vi "getPIDRawRead.vi"(11 "PIDController in":refnum<class "PIDController.lvclass">) -> (2 "PIDRawRead":dbl, 3 "PIDController out":refnum<class "PIDController.lvclass">)   [LabVIEW 2025, in "PIDController.lvclass"]
uses:
  PIDController.lvclass/PIDController.ctl
  PIDController.lvclass
panel:
  out "translatedPIDOutput":dbl
  in  "sensorValue":dbl
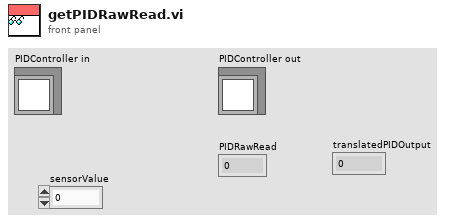
[diagram p1: front panel]
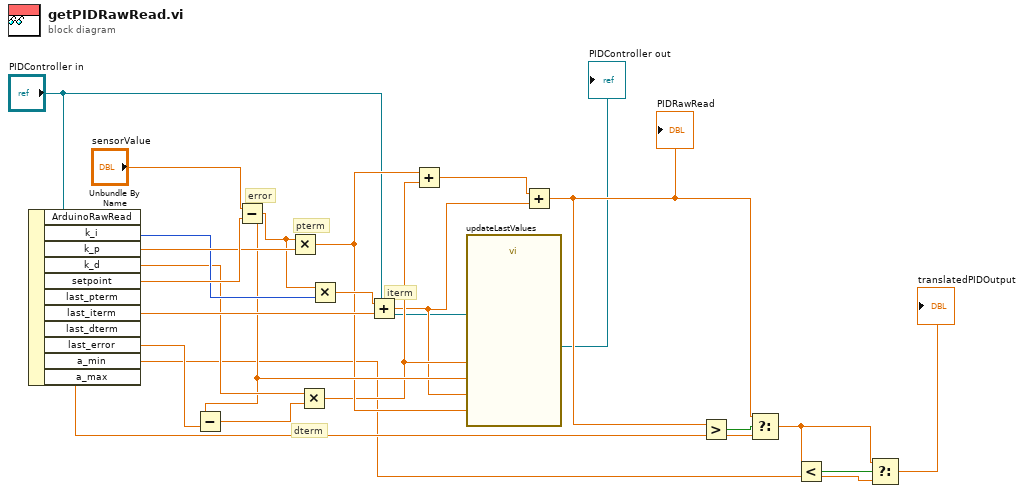
[diagram p0: block diagram]
diagram:
  # "dterm"
  # "iterm"
  # "error"
  # "pterm"
  n1 = Unbundle By Name("PIDController in") -> ("k_i"=w19:u16, "k_p"=w21:dbl, "k_d"=w17:dbl, "setpoint"=w22:dbl, "last_iterm"=w20:dbl, "last_error"=w15:dbl, "a_min"=w4:dbl, "a_max"=w7:dbl)  [unwired: 3 out]
  n2 = Subtract(x="sensorValue", y=w22) -> (x-y=w14:dbl)
  n3 = Subtract(x=w14, y=w15) -> (x-y=w16:dbl)
  n4 = Multiply(x=w14, y=w21) -> (x*y=w13:dbl)
  n5 = Multiply(x=w17, y=w16) -> (x*y=w12:dbl)
  n6 = Multiply(x=w14, y=w19) -> (x*y=w18:dbl)
  n7 = Add(x=w18, y=w20) -> (x+y=w11:dbl)
  n8 = Add(x=w13, y=w12) -> (x+y=w10:dbl)
  n9 = call "updateLastValues.vi"("last_iterm"=w11, "last_dterm"=w12, "last_error"=w14, "last_pterm"=w13, "PIDController in"="PIDController in") -> ("PIDController out"=→"PIDController out":refnum<class "PIDController.lvclass">)  [unwired: 5 in, 1 out]
  n10 = Add(x=w10, y=w11) -> (x+y=w8:dbl)
  "PIDRawRead" <- w8
  n11 = Greater?(x=w8, y=w7) -> (0:w9:bool)
  n12 = Select(t=w8, s=w9, f=w7) -> (s? t:f=w5:dbl)
  n13 = Less?(x=w5, y=w4) -> (x < y?=w6:bool)
  n14 = Select(t=w5, s=w6, f=w4) -> (s? t:f=→"translatedPIDOutput":dbl)
